vi "Read Stream from RT.vi"(10 "Connected notifier":refnum<notifier>, 11 "Message Queue in":refnum<class "Delacor_lib_QMH_Message Queue.lvclass">) -> (3 "Message Queue out":refnum<class "Delacor_lib_QMH_Message Queue.lvclass">)   [LabVIEW 2015, in "Tool Module.lvlib"]
uses:
  Tool Module.lvlib
  <vilib>/Delacor/Delacor QMH/Libraries/Message Queue_class/Delacor_lib_QMH_Message Queue.lvclass
  <vilib>/Delacor/Delacor QMH/Libraries/Message Queue_class/Delacor_lib_QMH_Enqueue Message (Single).vi
  Tool Interface/Tool Interface.lvlib
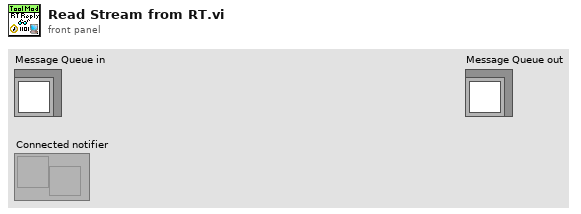
[diagram p1: front panel]
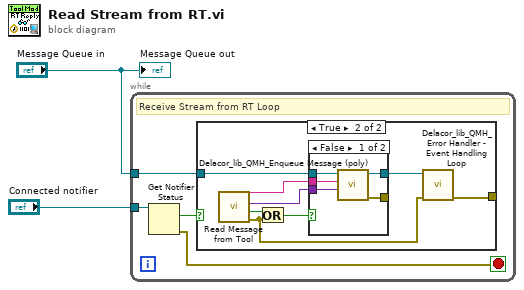
[diagram p0: block diagram]
diagram:
  n1 = while {
    tunnel: "Connected notifier" -> [w6]
    tunnel: "Message Queue in" -> [w4]
    stop <- w3 stop-if-true
    # "Receive Stream from RT Loop"
    n2 = Get Notifier Status(notifier=w6) -> (current notification=w5:bool, error out=w3:errorcluster)  [unwired: 1 in, 3 out]
    n3 = case shown="True" w5 {
      tunnel: w4 -> [_ w12]
      tunnel: [_ w7] -> _
      frame False {
      }
      frame True {
        n4 = call "Read Message from Tool.vi"() -> ("error out"=w8:errorcluster, "timed out?"=w14:bool, "Message Data"=w11:variant, "Message"=w10:string)  [unwired: 8 in]
        n5 = Or(x=w14, y=w8) -> (x .or. y?=w13:bool)
        n6 = case shown="False" w13 {
          tunnel: w12 -> [w19 w20]
          tunnel: w11 -> [w18 _]
          tunnel: w10 -> [w17 _]
          tunnel: [w16 w20] -> w9
          tunnel: [w15 _] -> _
          frame False {
            n7 = call-poly <vilib>:"Delacor_lib_QMH_Enqueue Message (poly).vi"("Message Data"=w18, "Message"=w17, "Message Queue in"=w19) -> ("error out"=w15:errorcluster, "Message Queue out"=w16:refnum<class "Delacor_lib_QMH_Message Queue.lvclass">)  [unwired: 7 in]
          }
          frame True {
          }
        }
        n8 = call-dynamic "Delacor_lib_QMH_Error Handler - Event Handling Loop.vi"("error in (no error)"=w8, "Message Queue in"=w9) -> ("dup error in"=w7:errorcluster)  [unwired: 8 in, 1 out]
      }
    }
  }
  "Message Queue out" <- "Message Queue in"
